vi "zadanie_na_ocene.vi"() -> ()   [LabVIEW 2025]
uses:
  <vilib>/measure/macond.llb/IIR Filter for 1 Chan.vi
  <vilib>/measure/NI_MAPro.lvlib
  <vilib>/Analysis/NI_AALPro.lvlib
  <vilib>/measure/NI_MABase.lvlib
panel:
  out "spektrum amplitudowe":waveform(dbl)[](graph)
  in  "signal type 3":T1(ring)
  in  "phase 3":dbl format="%.2p"
  in  "amplitude 3":dbl=1.0 format="%0.2p"
  in  "frequency 3":dbl=10.0 format="%0.2p"
  in  "signal type 2":T1(ring)
  in  "phase 2":dbl format="%.2p"
  in  "amplitude 2":dbl=1.0 format="%0.2p"
  in  "frequency 2":dbl=10.0 format="%0.2p"
  out "przebieg czasowy; biały - przed filtracją, czerwony - po":waveform(dbl)[](graph)
  in  "signal type":T1(ring)
  in  "phase":dbl format="%.2p"
  in  "amplitude":dbl=1.0 format="%0.2p"
  in  "frequency":dbl=10.0 format="%0.2p"
  out "widmo mocy; biały - przed filtracją, czerwony - po":waveform(dbl)[](graph)
  out "charakterystyka skokowa filtra":waveform(dbl)[](graph)
  in  "stop":bool
  out "charakterystyka fazowa filtra":cluster{"df":dbl, "df":dbl, "Phase H(w)":dbl[]}(graph)
  out "charakterystyka amplitudowa filtra":cluster{"f0":dbl, "df":dbl, "Mag H(w)":dbl[]}(graph)
  in  "IIR filter specifications":T2={"Topology"=enum."Butterworth", "Type"=enum."Lowpass", "Order"=1, "Lower Fc"=100.0, "Upper Fc"=200.0, "PB Ripple"=1.0, "SB Attenuation"=60.0} {"PB Ripple" format="%0.2f"; "SB Attenuation" format="%0.2f"; "Lower Fc" format="%0.2p"; "Upper Fc" format="%0.2p"}
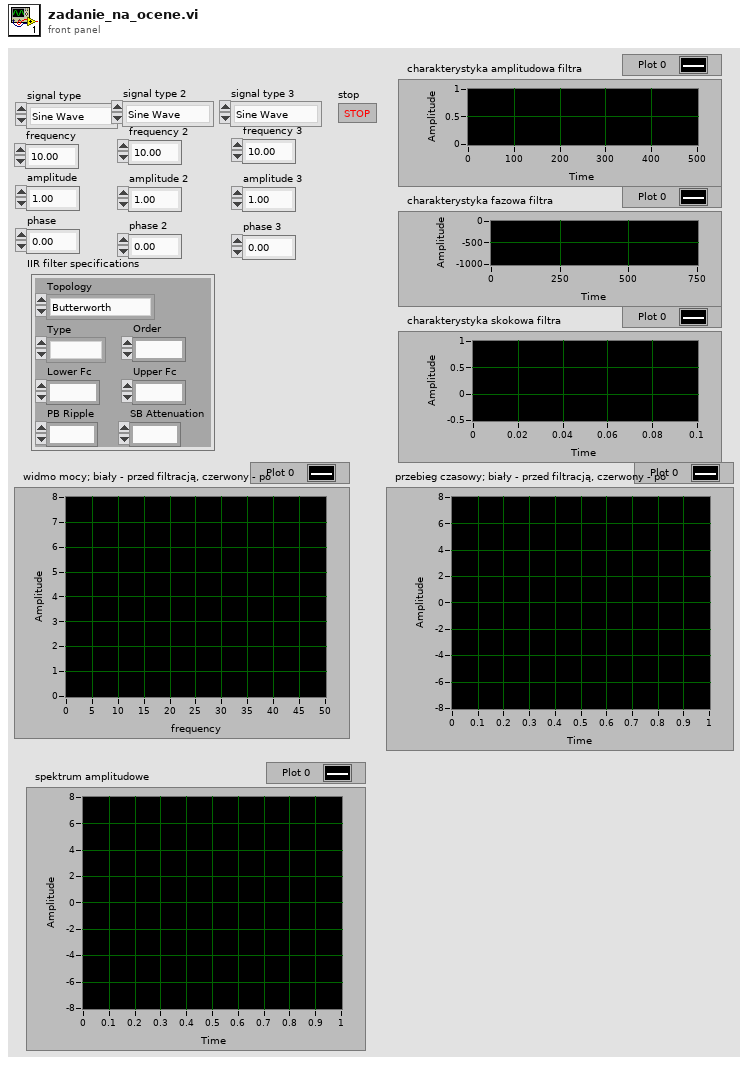
[diagram p1: front panel]
types:
  T1 = enum16{"Sine Wave", "Triangle Wave", "Square Wave", "Sawtooth Wave"}
  T2 = cluster{"Topology":enum16{"Off", "Butterworth", "Chebyshev", "Inverse Chebyshev", "Elliptic", "Bessel"}, "Type":enum16{"Lowpass", "Highpass", "Bandpass", "Bandstop"}, "Order":i32, "Lower Fc":dbl, "Upper Fc":dbl, "PB Ripple":dbl, "SB Attenuation":dbl}
  T3 = cluster{"magnitude H(w)":cluster{"f0":dbl, "df":dbl, "Mag H(w)":dbl[]}, "phase H(w)":cluster{"f0":dbl, "df":dbl, "Phase H(w)":dbl[]}, "order":i32}
  T4 = cluster{"df":dbl, "df":dbl, "Unwrapped Phase":dbl[]}
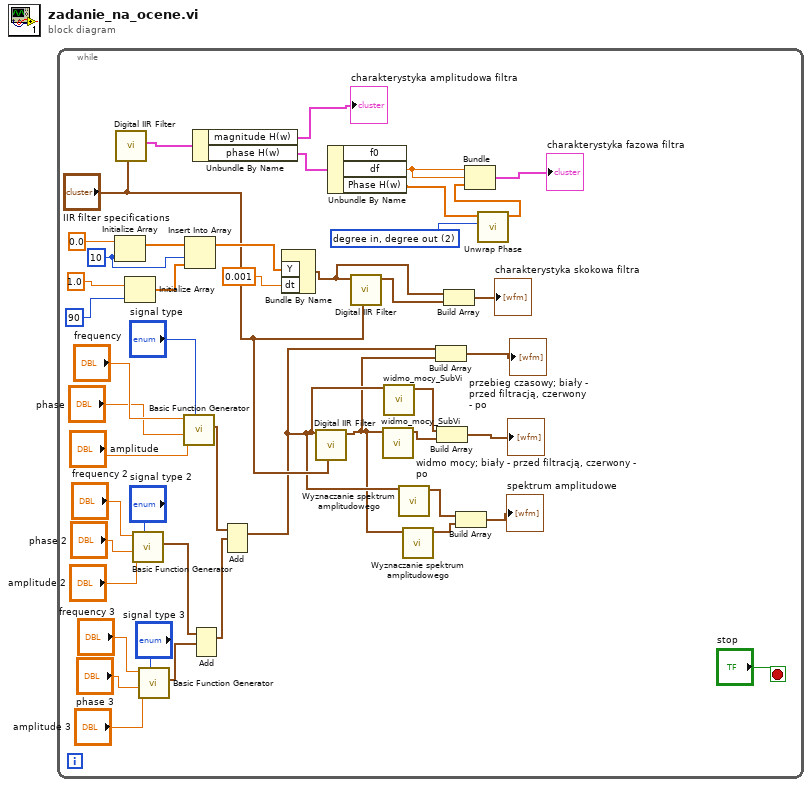
[diagram p0: block diagram]
diagram:
  n1 = while {
    stop <- "stop" stop-if-true
    w27 = 2 items=["radian in, radian out", "radian in, degree out", "degree in, degree out", "degree in, radian out"] ("phase unit")
    w34 = 10 ("dimension size")
    n2 = Initialize Array(0.0 ("element"), w34) -> (w36:dbl[])
    n3 = call-poly <vilib>:"Digital IIR Filter.vi"("IIR filter specifications"="IIR filter specifications") -> ("filter information"=w46:T3)  [unwired: 8 in, 2 out]
    n4 = Initialize Array(1.0 ("element"), 90 ("dimension size")) -> (w37:dbl[])
    n5 = call <vilib>:"Basic Function Generator.vi"("signal type"="signal type 2", "phase"="phase 2", "amplitude"="amplitude 2", "frequency"="frequency 2") -> ("signal out"=w9:waveform(dbl))  [unwired: 5 in, 2 out]
    n6 = call <vilib>:"Basic Function Generator.vi"("signal type"="signal type 3", "phase"="phase 3", "amplitude"="amplitude 3", "frequency"="frequency 3") -> ("signal out"=w8:waveform(dbl))  [unwired: 5 in, 2 out]
    n7 = call <vilib>:"Basic Function Generator.vi"("signal type"="signal type", "phase"="phase", "amplitude"="amplitude", "frequency"="frequency") -> ("signal out"=w7:waveform(dbl))  [unwired: 5 in, 2 out]
    n8 = Insert Into Array(array=w36, index=w34, new element=w37) -> (w38:dbl[])
    n9 = Add(1:w8, 2:w9) -> (0:w6:waveform(dbl))  [unwired: 1 in, 1 out]
    n10 = Unbundle By Name(w46) -> ("magnitude H(w)"=→"charakterystyka amplitudowa filtra":cluster{"f0":dbl, "df":dbl, "Mag H(w)":dbl[]}, "phase H(w)"=w45:cluster{"f0":dbl, "df":dbl, "Phase H(w)":dbl[]})
    n11 = Add(1:w6, 2:w7) -> (0:w2:waveform(dbl))  [unwired: 1 in, 1 out]
    n12 = Bundle By Name("Y"=w38, "dt"=0.001) -> (w30:waveform(dbl))  [unwired: 1 in]
    n13 = call-poly <vilib>:"Digital IIR Filter.vi"("IIR filter specifications"="IIR filter specifications", "signal in"=w2) -> ("signal out"=w1:waveform(dbl))  [unwired: 7 in, 2 out]
    n14 = Unbundle By Name(w45) -> ("df"=w44:dbl, "Phase H(w)"=w43:dbl[])  [unwired: 1 out]
    n15 = call-poly <vilib>:"Digital IIR Filter.vi"("IIR filter specifications"="IIR filter specifications", "signal in"=w30) -> ("signal out"=w29:waveform(dbl))  [unwired: 7 in, 2 out]
    n16 = call "widmo_mocy_SubVi.vi"("signal in"=w1) -> ("widmo mocy"=w25:waveform(dbl))  [unwired: 10 in]
    n17 = call "widmo_mocy_SubVi.vi"("signal in"=w2) -> ("widmo mocy"=w26:waveform(dbl))  [unwired: 10 in]
    n18 = call "Wyznaczanie spektrum amplitudowego.vi"("signal in"=w2) -> ("Waveform Graph"=w5:waveform(dbl))  [unwired: 4 in, 6 out]
    n19 = call "Wyznaczanie spektrum amplitudowego.vi"("signal in"=w1) -> ("Waveform Graph"=w4:waveform(dbl))  [unwired: 4 in, 6 out]
    n20 = Build Array(w2, w1) -> (→"przebieg czasowy; biały - przed filtracją, czerwony - po":waveform(dbl)[])
    n21 = Build Array(w26, w25) -> (→"widmo mocy; biały - przed filtracją, czerwony - po":waveform(dbl)[])
    n22 = Build Array(w30, w29) -> (→"charakterystyka skokowa filtra":waveform(dbl)[])
    n23 = Build Array(w5, w4) -> (→"spektrum amplitudowe":waveform(dbl)[])
    n24 = call <vilib>:"Unwrap Phase.vi"("phase unit"=w27, "Phase"=w43) -> ("Unwrapped Phase"=w40:dbl[])  [unwired: 8 in, 1 out]
    n25 = Bundle("df"=w44, "df"=w44, "Unwrapped Phase"=w40) -> (→"charakterystyka fazowa filtra":T4)  [unwired: 1 in]
  }
